vi "AerotechTrackLoop.vi"(0 "Gain [/s]":dbl, 3 "AEROTECH.TARGET":T2, 4 "Aerotech Position":dbl, 5 "Aerotech Time":timestamp, 7 "Track threshold":dbl) -> (1 "State":T1, 2 "Aerotech Velocity":dbl, 6 "Position error":dbl)   [LabVIEW 2009]
uses:
  Controls/AerotechTarget.ctl
  Controls/AerotechState.ctl
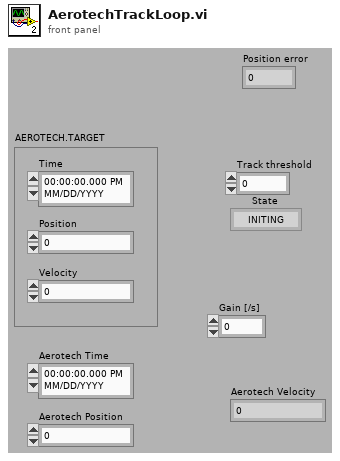
[diagram p1: front panel]
types:
  T1 = typedef "AerotechState.ctl" = enum16{"INITING", "IDLING", "SLEWING", "TRACKING", "MOVING", "HOMING", "STOPPING"}
  T2 = typedef "AerotechTarget.ctl" = cluster{"Time":timestamp, "Position":dbl, "Velocity":dbl}
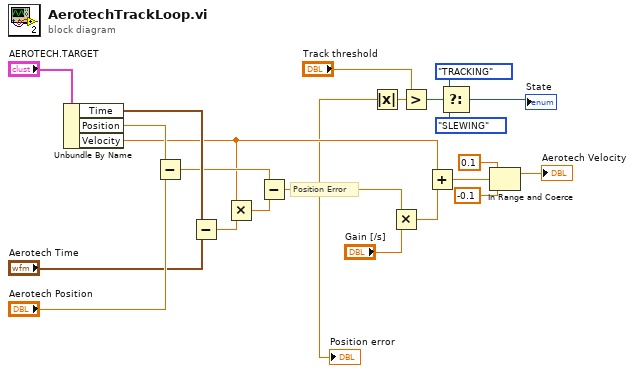
[diagram p0: block diagram]
diagram:
  # "Position Error"
  n1 = Unbundle By Name("AEROTECH.TARGET") -> ("Time"=w19:timestamp, "Position"=w21:dbl, "Velocity"=w12:dbl)
  n2 = Subtract(x=w21, y="Aerotech Position") -> (x-y=w16:dbl)
  n3 = Subtract(x=w19, y="Aerotech Time") -> (x-y=w17:dbl)
  n4 = Multiply(x=w12, y=w17) -> (x*y=w15:dbl)
  n5 = Subtract(x=w16, y=w15) -> (x-y=w6:dbl)
  "Position error" <- w6
  n6 = Absolute Value(x=w6) -> (abs(x)=w5:dbl)
  n7 = Multiply(x=w6, y="Gain [/s]") -> (x*y=w13:dbl)
  n8 = Greater?(x="Track threshold", y=w5) -> (0:w10:bool)
  n9 = Add(x=w12, y=w13) -> (x+y=w4:dbl)
  n10 = Select(t=AerotechState."TRACKING" ("State"), s=w10, f=AerotechState."SLEWING" ("State")) -> (s? t:f=→"State":T1)
  n11 = In Range and Coerce(upper limit=0.1, x=w4, lower limit=-0.1) -> (coerced(x)=→"Aerotech Velocity":dbl)  [unwired: 1 out]
